vi "Image FFT line by line with conv to time from lambda.vi"(10 "Input image 2":u16[][](graph), 11 "File Path":path=path "C:/Users/tony/Documents/Tony Labview SVN/LBL data analysis/test data/Scan013_TS-ChromexCam_147.png") -> ()   [LabVIEW 2013]
panel:
  in  "Zero padding":cluster{"zero pad":bool, "# Zeros":i32}={"zero pad"=FALSE, "# Zeros"=10000}
  in  "Time Chop":T1={"Chop!"=FALSE, "min time"=5e-13, "max time"=1.3e-12} {"max time" format="%#_6p"; "min time" format="%#_6p"}
  in  "Tab Control":T2(tab)
  in  "calibration":T3={"start index"=470, "length"=50, "Cal array"=[775.3345, 0.046953, 0.0]}
  in  "Cut?":bool=TRUE
  in  "color table MS 2":u32[](array[colorbox])=[0, 79, 65873, 197460, 263254, 394840, 460635, 526429, 658015, 723810, 789860, 921190, 986984, 1118571, 1184365, 1250415, 1381746, 1447540, 1513590, 1644921, 1710715, 1842301, 1908096, 1974146, 2105476, 2171271, 2237321, 2368651, 2434702, 2566032, 2631826, 2697876, 2829207, 2895257, 2961051, 3092382, 3158432, 3289762, 3355813, 3421607, 3552937, 3618988, 3750318, 3816368, 3882163, 4013493, 4079543, 4145338, 4276668, 4342718, 4474048, 4540099, 4605893, 4737223, 4803274, 4869068, 5000654, 5066449, 5197779, 5263829, 5329624, 5461210, 5527004, 5592799, 5724385, 5790179, 5921766, 5987560, 6053354, 6184940, 6250735, 6316785, 6448115, 6513910, 6645496, 6711290, 6777341, 6908671, 6974462, 7106044, 7171835, 7237625, 7369208, 7434998, 7501045, 7632371, 7698162, 7829745, 7895535, 7961582, 8092908, 8158699, 8224745, 8356072, 8422119, 8553445, 8619236, 8685282, 8816609, 8882655, 8948446, 9079772, 9145819, 9277146, 9343192, 9408983, 9540309, 9606356, 9672146, 9803473, 9869519, 10000846, 10066893, 10132683, 10264010, 10330056, 10461383, 10527429, 10593220, 10724546, 10790593, 10856384, 10987966, 11053757, 11185083, 11251130, 11316920, 11448503, 11514294, 11580084, 11711667, 11777457, 11909040, 11974830, 12040621, 12172203, 12237994, 12304041, 12435367, 12501158, 12632740, 12698531, 12764321, 12895904, 12961694, 13027741, 13159068, 13224858, 13356441, 13422231, 13488278, 13619604, 13685395, 13816978, 13882768, 13948815, 14080141, 14145932, 14211978, 14343305, 14409351, 14540678, 14606469, 14672515, 14803842, 14869888, 14935679, 15067005, 15133052, 15264378, 15330169, 15396216, 15527542, 15593589, 15659379, 15790706, 15856752, 15988079, 16054125, 16119916, 16251243, 16317289, 16383080, 16514662, 16580453, 16710499, 16775266, 16774241, 16773215, 16772446, 16771420, 16770651, 16769625, 16768600, 16767830, 16766805, 16765780, 16765010, 16763985, 16762959, 16762190, 16761164, 16760139, 16759369, 16758344, 16757319, 16756549, 16755524, 16754754, 16753729, 16752703, 16751934, 16750909, 16749883, 16749114, 16748088, 16747063, 16746293, 16745268, 16744498, 16743473, 16742448, 16741678, 16740653, 16739627, 16738858, 16737832, 16736807, 16736037, 16735012, 16733987, 16733217, 16732192, 16731166, 16730397, 16729371, 16728602, 16727576, 16726551, 16725782, 16724756, 16723731, 16722961, 16721936, 16720910, 16720141, 16719116, 16718346, 16717321, 16716295, 16715526, 16714500, 16713475, 16712705, 0, 0]
  out "Input image":u16[][](graph)
  out "cut image":u16[][](graph)
  out "FFT of image (line by line)":dbl[][](graph)
  out "FFT line by line normalized":dbl[][](graph)
  out "FFT of input spectrum 3":T4(graph) caption="Lineout graph"
  out "FFT of input spectrum 4":T5(graph) caption="Lineout graph"
  # "offset\n\ngrad\n\nquad"
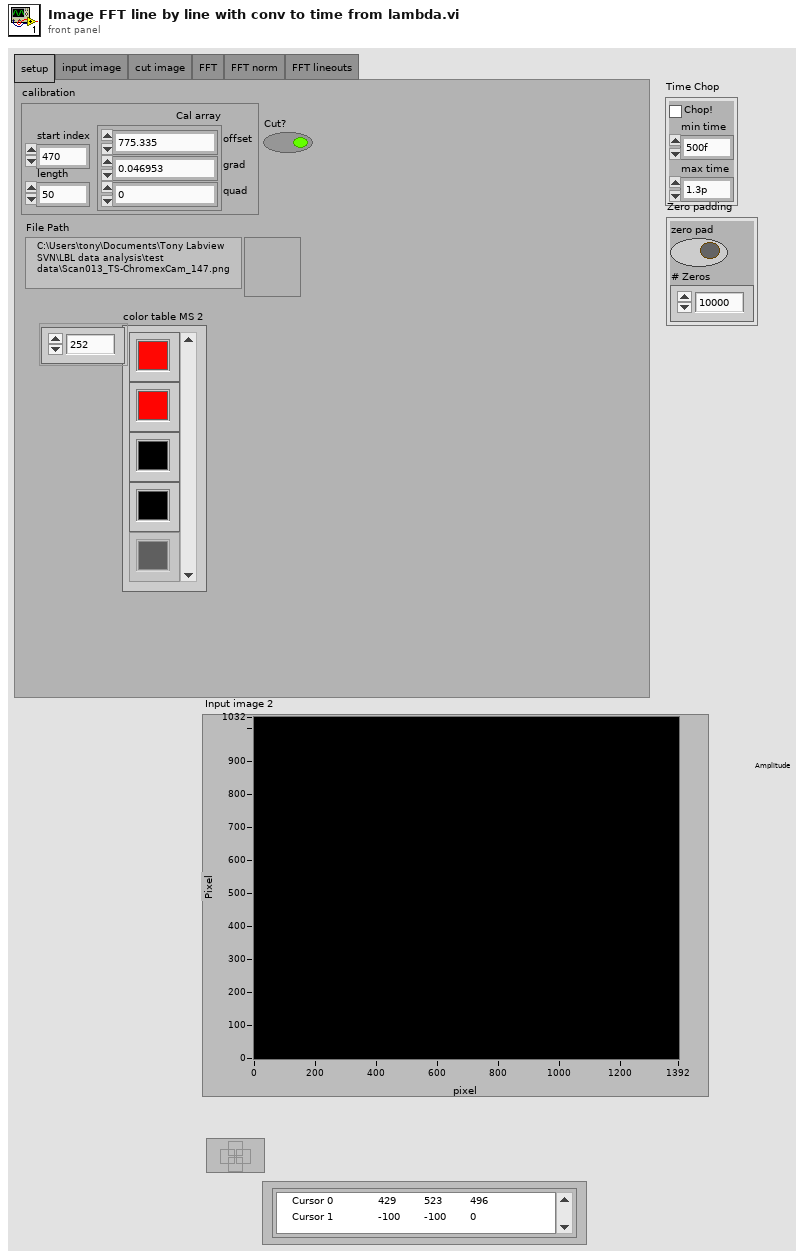
[diagram p1: front panel]
types:
  T1 = cluster{"Chop!":bool, "min time":sgl, "max time":sgl}
  T2 = enum32{"setup", "input image", "cut image", "FFT", "FFT norm", "FFT lineouts"}
  T3 = cluster{"start index":i32, "length":i32, "Cal array":dbl[]}
  T4 = cluster{"y_cut":dbl[], "Best Gaussian Fit":dbl[]}[]
  T5 = cluster{"Ramp Pattern":dbl[], "Amp Spectrum Mag (Vrms)":dbl[]}
  T6 = cluster{"Wavelength Array":dbl[], "Input image 2":u16[]}
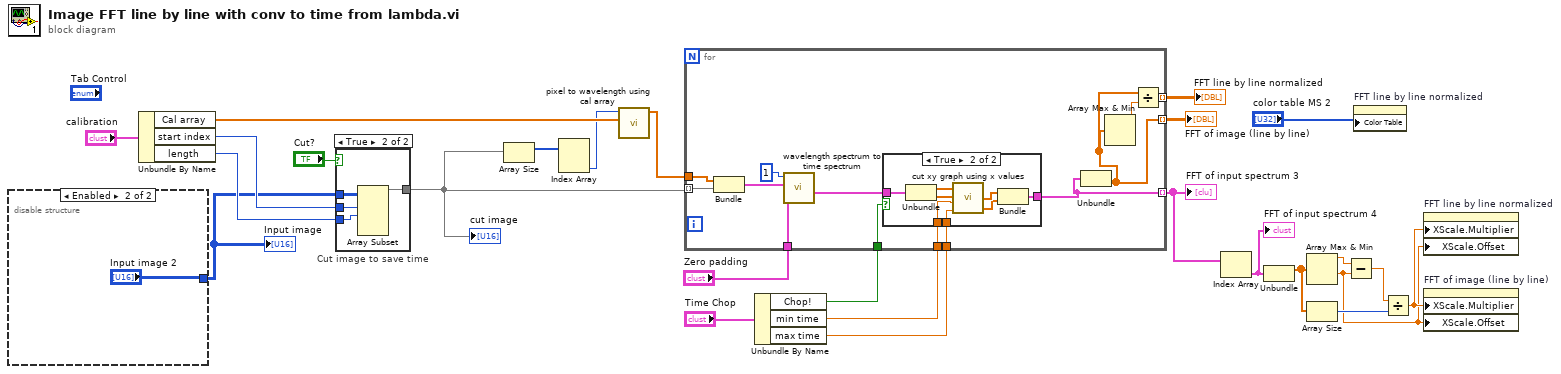
[diagram p0: block diagram]
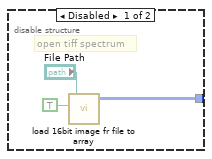
[diagram p2: hidden frame]
diagram:
  n1 = disable-structure shown="Enabled" {
    disable-tunnel: [w27 "Input image 2"] -> w1
    frame Disabled {
      # "open tiff spectrum"
      n2 = call "load 16bit image fr file to array.vi"("Dispose images"=TRUE, "File Path"="File Path") -> ("Intensity Graph"=w27:u16[][])  [unwired: 2 in, 2 out]
    }
    frame Enabled {
    }
  }
  "Input image" <- w1
  n3 = Unbundle By Name("calibration") -> ("Cal array"=w26:dbl[], "start index"=w23:i32, "length"=w22:i32)
  n4 = case "Cut image to save time" shown="True" "Cut?" {
    tunnel: w1 -> [w31 w35]
    tunnel: [w31 w34] -> w20
    tunnel: w23 -> [_ w33]
    tunnel: w22 -> [_ w32]
    frame False {
    }
    frame True {
      n5 = Array Subset(array=w35, index (row)=w33, length (row)=w32) -> (w34:u16[][])  [unwired: 2 in]
    }
  }
  "cut image" <- w20
  n6 = Array Size(array=w20) -> (size(s)=w19:i32[])
  n7 = Index Array(array=w19) -> (element #2=w18:i32)  [unwired: 2 in, 1 out]
  n8 = call "pixel to wavelength using cal array.vi"("Cal array"=w26, "# pix"=w18) -> ("Wavelength Array"=w17:dbl[])  [unwired: 9 in]
  n9 = Unbundle By Name("Time Chop") -> ("Chop!"=w12:bool, "min time"=w11:sgl, "max time"=w10:sgl)
  n10 = for {
    tunnel: w17 -> [w48]
    tunnel: w20 -> [w47] mode=indexing
    tunnel: [w36] -> w15 mode=indexing
    tunnel: [w43] -> w21 mode=indexing
    tunnel: [w42] -> w16 mode=indexing
    tunnel: "Zero padding" -> [w41]
    tunnel: w12 -> [w39]
    tunnel: w11 -> [w38]
    tunnel: w10 -> [w37]
    n11 = Bundle("Wavelength Array"=w48, "Input image 2"=w47) -> (w46:T6)  [unwired: 1 out]
    n12 = call "wavelength spectrum to time spectrum.vi"("Zero padding"=w41, "Input spectrum (nm)"=w46, "# interpolated points / # original points"=1) -> ("FFT of input spectrum"=w40:T5)  [unwired: 5 in, 3 out]
    n13 = case shown="True" w39 {
      tunnel: w40 -> [w49 w57]
      tunnel: w38 -> [_ w54]
      tunnel: w37 -> [_ w53]
      tunnel: [w49 w50] -> w36
      frame False {
      }
      frame True {
        n14 = Unbundle(w57) -> ("Ramp Pattern"=w56:dbl[], "Amp Spectrum Mag (Vrms)"=w55:dbl[])
        n15 = call "cut xy graph using x values.vi"("x_max"=w53, "x_min"=w54, "f(x)"=w55, "x"=w56) -> ("y_cut"=w51:dbl[], "x_cut"=w52:dbl[])  [unwired: 1 out]
        n16 = Bundle("x_cut"=w52, "y_cut"=w51) -> (w50:cluster{"x_cut":dbl[], "y_cut":dbl[]})  [unwired: 1 in]
      }
    }
    n17 = Unbundle(w36) -> ("y_cut"=w43:dbl[])  [unwired: 1 out]
    n18 = Array Max & Min(array=w43) -> (max value=w44:dbl)  [unwired: 3 out]
    n19 = Divide(x=w43, y=w44) -> (x/y=w42:dbl[])
  }
  "FFT of image (line by line)" <- w21
  "FFT of input spectrum 3" <- w15
  "FFT line by line normalized" <- w16
  n20 = Index Array(array=w15) -> (element=w8:cluster{"x_cut":dbl[], "y_cut":dbl[]})  [unwired: 1 in]
  "FFT of input spectrum 4" <- w8
  n21 = Unbundle(w8) -> ("x_cut"=w7:dbl[])  [unwired: 1 out]
  n22 = Array Max & Min(array=w7) -> (max value=w5:dbl, min value=w2:dbl)  [unwired: 2 out]
  n23 = Array Size(array=w7) -> (size(s)=w6:i32)
  n24 = Subtract(x=w5, y=w2) -> (x-y=w4:dbl)
  n25 = property on="FFT line by line normalized" class="IntGraph (strict)"("Color Table"="color table MS 2") -> ()  [unwired: 2 in, 2 out]
  n26 = Divide(x=w4, y=w6) -> (x/y=w3:dbl)
  n27 = property on="FFT line by line normalized" class="IntGraph (strict)"("XScale.Multiplier"=w3, "XScale.Offset"=w2) -> ()  [unwired: 2 in, 2 out]
  n28 = property on="FFT of image (line by line)" class="IntGraph (strict)"("XScale.Multiplier"=w3, "XScale.Offset"=w2) -> ()  [unwired: 2 in, 2 out]
